vi "Stop Acquisition.vi"(8 "error in (no error)":errorcluster, 11 "Hardware Resources in":T1) -> (0 "error out":errorcluster)   [LabVIEW 2014, in "Flicker.lvlib" / "Flicker Acquisition.lvlib"]
doc: "Stops the acquisition."
uses:
  Flicker Acquisition.lvlib
  Hardware Configuration.ctl
  Signal Type.ctl
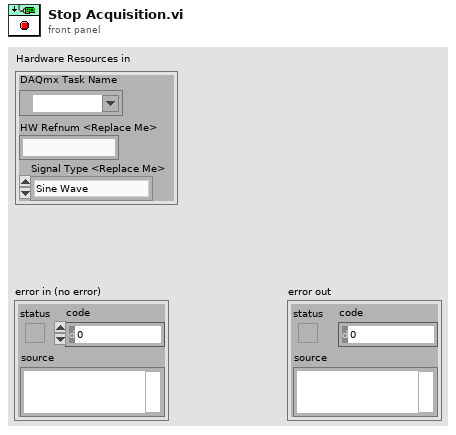
[diagram p1: front panel]
types:
  T1 = typedef "Flicker.lvlib/Flicker Acquisition.lvlib/Hardware Configuration.ctl" = cluster{"DAQmx Task Name":refnum<k21>, "HW Refnum <Replace Me>":string, "Signal Type <Replace Me>":T2}
  T2 = typedef "Flicker.lvlib/Flicker Acquisition.lvlib/Signal Type.ctl" = enum16{"Sine Wave", "Square with Noise"}
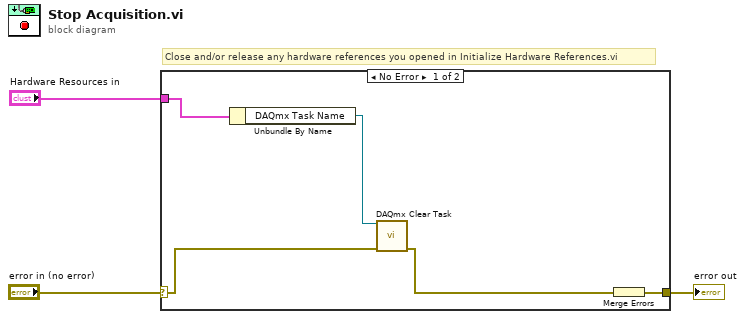
[diagram p0: block diagram]
diagram:
  # "Close and/or release any hardware references you opened in Initialize Hardware References.vi"
  n1 = case shown="No Error" "error in (no error)" {
    selector: "error in (no error)" -> [w6 w9]
    tunnel: [w8 w9] -> w2
    tunnel: "Hardware Resources in" -> [w7 _]
    frame No Error {
      n2 = Unbundle By Name(w7) -> ("DAQmx Task Name"=w4:refnum<k21>)
      n3 = call <vilib>:"DAQmx Clear Task.vi"("task in"=w4, "error in"=w6) -> ("error out"=w5:errorcluster)  [unwired: 13 in]
      n4 = Merge Errors(w5) -> (w8:errorcluster)
    }
    frame Error {
    }
  }
  "error out" <- w2
